vi "Write Sub Panel Monedas.vi"(8 "error in (no error)":errorcluster, 10 "Sub Panel Monedas":refnum<vi>, 11 "Quetzal Actor in":refnum<class "Quetzal Actor.lvclass">) -> (0 "error out":errorcluster, 3 "Quetzal Actor out":refnum<class "Quetzal Actor.lvclass">)   [LabVIEW 2020, in "Quetzal Actor.lvlib" / "Quetzal Actor.lvclass"]
uses:
  Quetzal Actor.lvclass
  Quetzal Actor.lvclass/Quetzal Actor.ctl
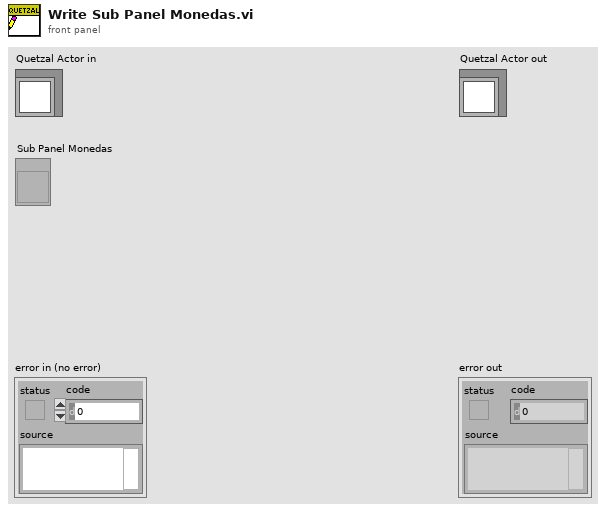
[diagram p1: front panel]
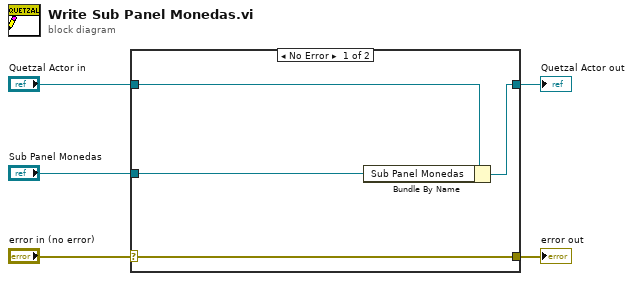
[diagram p0: block diagram]
diagram:
  n1 = case shown="No Error" "error in (no error)" {
    selector: "error in (no error)" -> [w9 w10]
    tunnel: [w9 w10] -> w4
    tunnel: [w7 w11] -> w2
    tunnel: "Quetzal Actor in" -> [w8 w11]
    tunnel: "Sub Panel Monedas" -> [w6 _]
    frame No Error {
      n2 = Bundle By Name(cluster=w8, "Sub Panel Monedas"=w6) -> (w7:refnum<class "Quetzal Actor.lvclass">)
    }
    frame Error {
    }
  }
  "error out" <- w4
  "Quetzal Actor out" <- w2
